vi "Write.vi"(7 "length":u16, 8 "error in (no error)":errorcluster, 9 "Start address":string, 10 "Read Type":variant, 11 "MelsecTCP in":refnum<class "Inovance5UTcp.lvclass">) -> (0 "error out":errorcluster, 3 "MelsecTCP out":refnum<class "Inovance5UTcp.lvclass">)   [LabVIEW 2020, in "HslCommunication.lvlib" / "Inovance5UTcp.lvclass"]
uses:
  Inovance5UTcp.lvclass
  C:/Users/Fred Guo/Desktop/API_Salcomp_CMES/Libraries/HslCommunication/HslCommunication.dll
  HslCommunication.dll
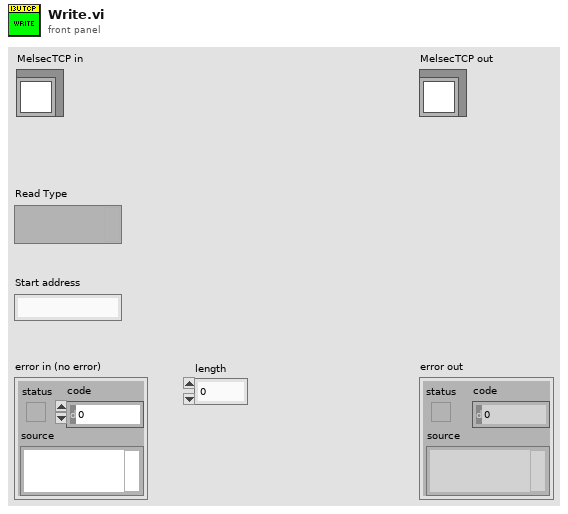
[diagram p1: front panel]
types:
  T1 = typedef "Type Descriptor Enumeration__ogtk.ctl" = enum8{"<Null>", "I8", "I16", "I32", "I64", "U8", "U16", "U32", "U64", "SGL", "DBL", "EXT", "CSG", "CDB", "CXT", "0x0F", "0x10", "0x11", "0x12", "0x13", "0x14", "Enum U8", "Enum U16", "Enum U32", "Enum U64", "SGL PQ", "DBL PQ", "EXT PQ", "CSG PQ", "CDB PQ", "CXT PQ", "0x1F", "0x20", "Boolean", "0x22", "0x23", "0x24", "0x25", "0x26", "0x27", "0x28", "0x29", "0x2A", "0x2B", "0x2C", "0x2D", "0x2E", "0x2F", "String", "0x31", "Path", "Pict", "0x34", "0x35", "0x36", "DAQ", "0x38", "0x39", "0x3A", "0x3B", "0x3C", "0x3D", "0x3E", "0x3F", "Array", "0x41", "0x42", "0x43", "0x44", "0x45", "0x46", "0x47", "0x48", "0x49", "0x4A", "0x4B", "0x4C", "0x4D", "0x4E", "0x4F", "Cluster", "0x51", "0x52", "Variant", "Waveform", "0x55", "0x56", "0x57", "0x58", "0x59", "0x5A", "0x5B", "0x5C", "0x5D", "0x5E", "Fixed Point", "0x60", "0x61", "0x62", "0x63", "0x64", "0x65", "0x66", "0x67", "0x68", "0x69", "0x6A", "0x6B", "0x6C", "0x6D", "0x6E", "0x6F", "Refnum", "0x71", "0x72", "Set Collection", "Map Collection"}
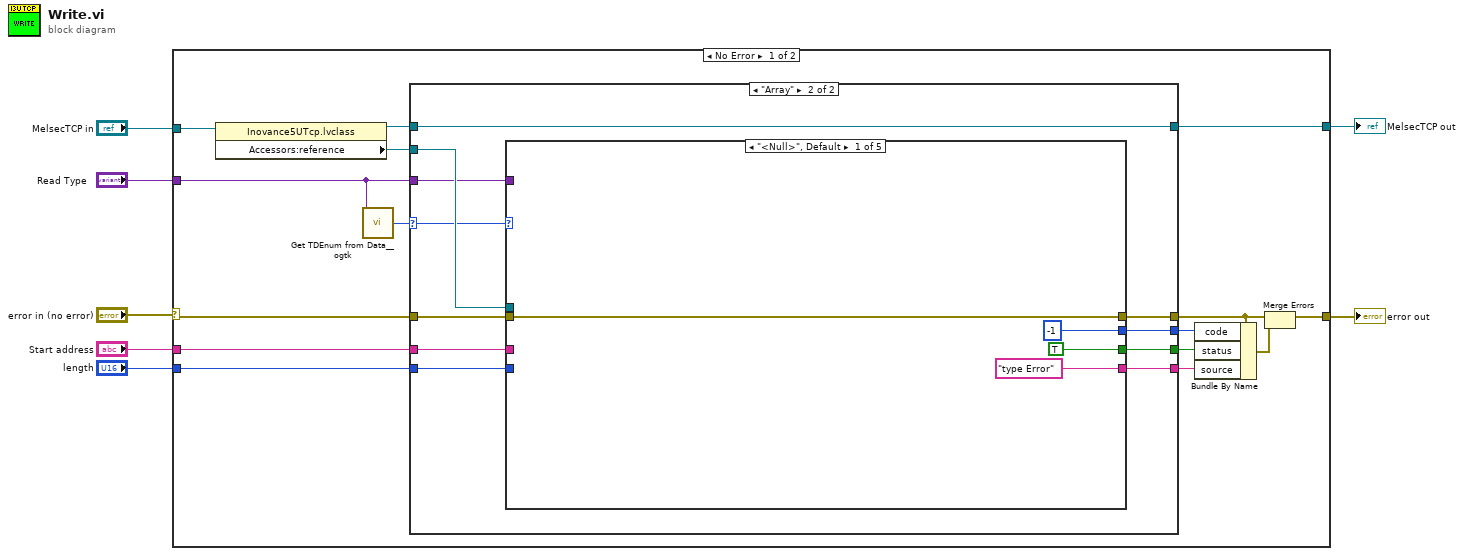
[diagram p0: block diagram]
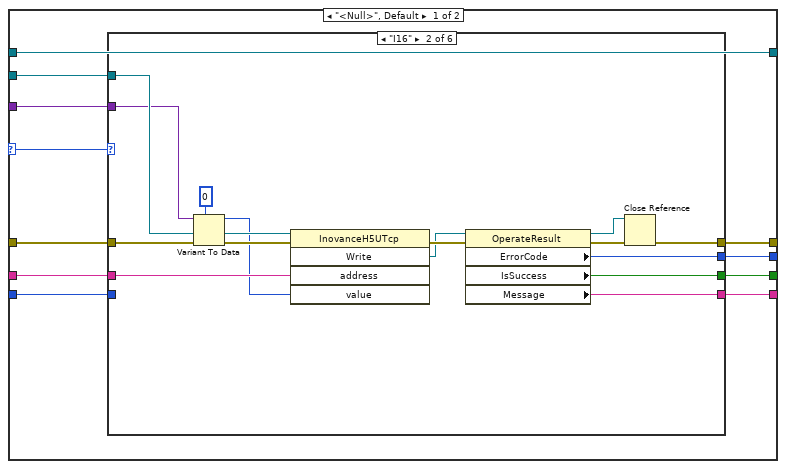
[diagram p2: hidden frame]
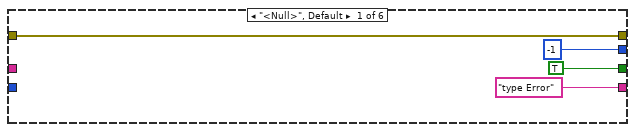
[diagram p3: hidden frame]
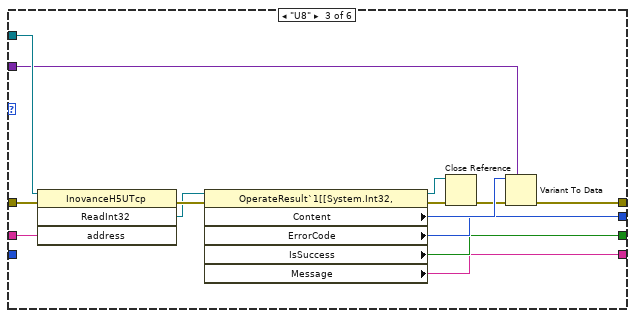
[diagram p4: hidden frame]
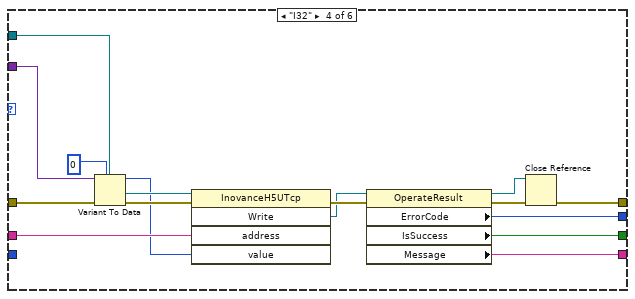
[diagram p5: hidden frame]
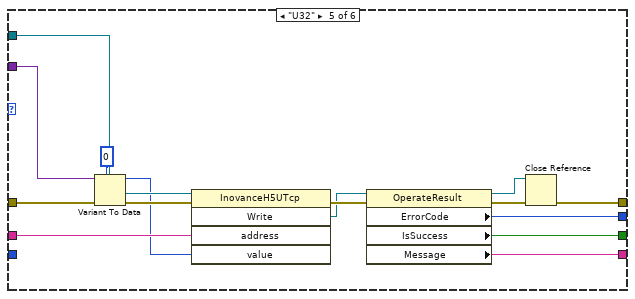
[diagram p6: hidden frame]
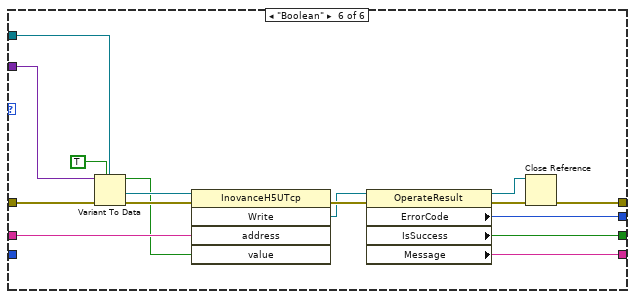
[diagram p7: hidden frame]
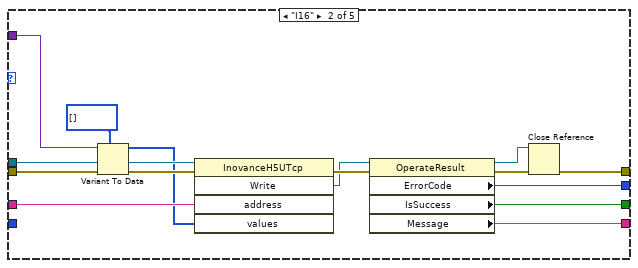
[diagram p8: hidden frame]
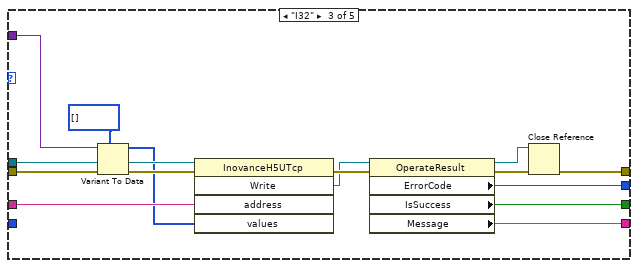
[diagram p9: hidden frame]
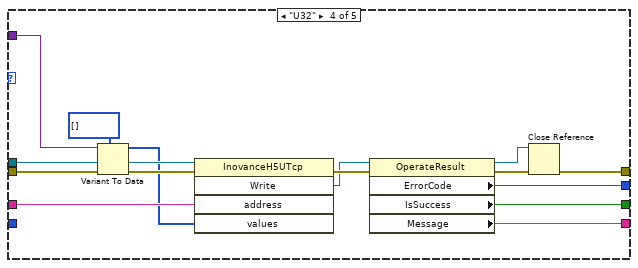
[diagram p10: hidden frame]
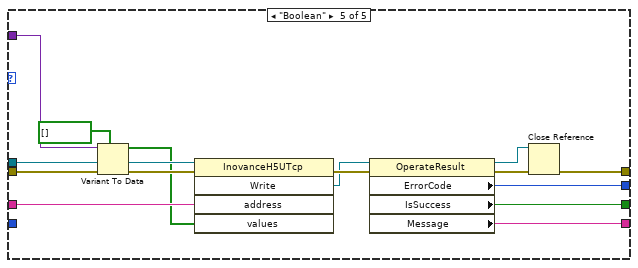
[diagram p11: hidden frame]
diagram:
  n1 = case shown="No Error" "error in (no error)" {
    selector: "error in (no error)" -> [w18 w188]
    tunnel: "MelsecTCP in" -> [w22 w187]
    tunnel: [w8 w187] -> w7
    tunnel: "Start address" -> [w20 _]
    tunnel: [w15 w188] -> w2
    tunnel: "length" -> [w19 _]
    tunnel: "Read Type" -> [w17 _]
    frame No Error {
      n2 = property class="Inovance5UTcp.lvclass"(reference=w22) -> (reference out=w9:refnum<class "Inovance5UTcp.lvclass">, "Accessors:reference"=w21:refnum<k24>)  [unwired: 1 in, 1 out]
      n3 = call <userlib>:"Get TDEnum from Data__ogtk.vi"("Data"=w17) -> ("Type Descriptor Enumeration"=w16:T1)  [unwired: 4 in]
      n4 = case shown="\"Array\"" w16 {
        selector: w16 -> [w27 w116]
        tunnel: w21 -> [w33 w122]
        tunnel: w20 -> [w32 w121]
        tunnel: w19 -> [w31 w120]
        tunnel: w18 -> [w28 w117]
        tunnel: [w30 w119] -> w11
        tunnel: w17 -> [w29 w118]
        tunnel: [w26 w115] -> w14
        tunnel: [w24 w113] -> w12
        tunnel: [w25 w114] -> w13
        tunnel: [w23 w112] -> w8
        tunnel: w9 -> [w23 w112]
        frame "<Null>", Default {
          n5 = case shown="\"I16\"" w27 {
            tunnel: w33 -> [_ w42 w66 w71 w86 w101]
            tunnel: w32 -> [_ w52 w65 w81 w96 w111]
            tunnel: w31 -> [_ _ _ _ _ _]
            tunnel: w28 -> [w37 w51 w64 w80 w95 w110]
            tunnel: [w37 w46 w57 w75 w90 w105] -> w30
            tunnel: [-1 ("ErrorCode") w45 w56 w74 w89 w104] -> w26
            tunnel: [TRUE ("IsSuccess") w44 w55 w73 w88 w103] -> w25
            tunnel: ["type Error" ("Message") w43 w54 w72 w87 w102] -> w24
            tunnel: w29 -> [_ w40 w53 w69 w84 w99]
            frame "<Null>", Default {
            }
            frame "I16" {
              n6 = Variant To Data(error in=w51, type=i16 0, Variant=w40) -> (data=w38:i16, error out=w41:errorcluster)
              n7 = invoke class="InovanceH5UTcp" method="Write"(reference=w42, error in=w41, "address"=w52, "value"=w38) -> (error out=w50:errorcluster, "Write"=w48:refnum<k24>)  [unwired: 1 in, 3 out]
              n8 = property class="OperateResult"(reference=w48, error in=w50) -> (reference out=w47:refnum<k24>, error out=w49:errorcluster, "ErrorCode"=w45:i32, "IsSuccess"=w44:bool, "Message"=w43:string)
              n9 = Close Reference(reference=w47, error in (no error)=w49) -> (error out=w46:errorcluster)
            }
            frame "U8" {
              n10 = invoke class="InovanceH5UTcp" method="ReadInt32"(reference=w66, error in=w64, "address"=w65) -> (error out=w63:errorcluster, "ReadInt32"=w61:refnum<k24>)  [unwired: 1 in, 2 out]
              n11 = property class="OperateResult`1[[System.Int32, "(reference=w61, error in=w63) -> (reference out=w60:refnum<k24>, error out=w62:errorcluster, "Content"=w59:i32, "ErrorCode"=w56:i32, "IsSuccess"=w55:bool, "Message"=w54:string)
              n12 = Close Reference(reference=w60, error in (no error)=w62) -> (error out=w58:errorcluster)
              n13 = Variant To Data(error in=w58, type=w53, Variant=w59) -> (error out=w57:errorcluster)  [unwired: 1 out]
            }
            frame "I32" {
              n14 = Variant To Data(error in=w80, type=0, Variant=w69) -> (data=w67:i32, error out=w70:errorcluster)
              n15 = invoke class="InovanceH5UTcp" method="Write"(reference=w71, error in=w70, "address"=w81, "value"=w67) -> (error out=w79:errorcluster, "Write"=w77:refnum<k24>)  [unwired: 1 in, 3 out]
              n16 = property class="OperateResult"(reference=w77, error in=w79) -> (reference out=w76:refnum<k24>, error out=w78:errorcluster, "ErrorCode"=w74:i32, "IsSuccess"=w73:bool, "Message"=w72:string)
              n17 = Close Reference(reference=w76, error in (no error)=w78) -> (error out=w75:errorcluster)
            }
            frame "U32" {
              n18 = Variant To Data(error in=w95, type=u32 0, Variant=w84) -> (data=w82:u32, error out=w85:errorcluster)
              n19 = invoke class="InovanceH5UTcp" method="Write"(reference=w86, error in=w85, "address"=w96, "value"=w82) -> (error out=w94:errorcluster, "Write"=w92:refnum<k24>)  [unwired: 1 in, 3 out]
              n20 = property class="OperateResult"(reference=w92, error in=w94) -> (reference out=w91:refnum<k24>, error out=w93:errorcluster, "ErrorCode"=w89:i32, "IsSuccess"=w88:bool, "Message"=w87:string)
              n21 = Close Reference(reference=w91, error in (no error)=w93) -> (error out=w90:errorcluster)
            }
            frame "Boolean" {
              n22 = Variant To Data(error in=w110, type=TRUE, Variant=w99) -> (data=w97:bool, error out=w100:errorcluster)
              n23 = invoke class="InovanceH5UTcp" method="Write"(reference=w101, error in=w100, "address"=w111, "value"=w97) -> (error out=w109:errorcluster, "Write"=w107:refnum<k24>)  [unwired: 1 in, 3 out]
              n24 = property class="OperateResult"(reference=w107, error in=w109) -> (reference out=w106:refnum<k24>, error out=w108:errorcluster, "ErrorCode"=w104:i32, "IsSuccess"=w103:bool, "Message"=w102:string)
              n25 = Close Reference(reference=w106, error in (no error)=w108) -> (error out=w105:errorcluster)
            }
          }
        }
        frame "Array" {
          n26 = case shown="\"<Null>\", Default" w116 {
            tunnel: w122 -> [_ w131 w146 w161 w176]
            tunnel: w121 -> [_ w141 w156 w171 w186]
            tunnel: w120 -> [_ _ _ _ _]
            tunnel: w117 -> [w126 w140 w155 w170 w185]
            tunnel: [w126 w135 w150 w165 w180] -> w119
            tunnel: [-1 ("ErrorCode") w134 w149 w164 w179] -> w115
            tunnel: [TRUE ("IsSuccess") w133 w148 w163 w178] -> w114
            tunnel: ["type Error" ("Message") w132 w147 w162 w177] -> w113
            tunnel: w118 -> [_ w129 w144 w159 w174]
            frame "<Null>", Default {
            }
            frame "I16" {
              n27 = Variant To Data(error in=w140, type=i16[] [], Variant=w129) -> (data=w127:i16[], error out=w130:errorcluster)
              n28 = invoke class="InovanceH5UTcp" method="Write"(reference=w131, error in=w130, "address"=w141, "values"=w127) -> (error out=w139:errorcluster, "Write"=w137:refnum<k24>)  [unwired: 1 in, 3 out]
              n29 = property class="OperateResult"(reference=w137, error in=w139) -> (reference out=w136:refnum<k24>, error out=w138:errorcluster, "ErrorCode"=w134:i32, "IsSuccess"=w133:bool, "Message"=w132:string)
              n30 = Close Reference(reference=w136, error in (no error)=w138) -> (error out=w135:errorcluster)
            }
            frame "I32" {
              n31 = Variant To Data(error in=w155, type=i32[] [], Variant=w144) -> (data=w142:i32[], error out=w145:errorcluster)
              n32 = invoke class="InovanceH5UTcp" method="Write"(reference=w146, error in=w145, "address"=w156, "values"=w142) -> (error out=w154:errorcluster, "Write"=w152:refnum<k24>)  [unwired: 1 in, 3 out]
              n33 = property class="OperateResult"(reference=w152, error in=w154) -> (reference out=w151:refnum<k24>, error out=w153:errorcluster, "ErrorCode"=w149:i32, "IsSuccess"=w148:bool, "Message"=w147:string)
              n34 = Close Reference(reference=w151, error in (no error)=w153) -> (error out=w150:errorcluster)
            }
            frame "U32" {
              n35 = Variant To Data(error in=w170, type=u32[] [], Variant=w159) -> (data=w157:u32[], error out=w160:errorcluster)
              n36 = invoke class="InovanceH5UTcp" method="Write"(reference=w161, error in=w160, "address"=w171, "values"=w157) -> (error out=w169:errorcluster, "Write"=w167:refnum<k24>)  [unwired: 1 in, 3 out]
              n37 = property class="OperateResult"(reference=w167, error in=w169) -> (reference out=w166:refnum<k24>, error out=w168:errorcluster, "ErrorCode"=w164:i32, "IsSuccess"=w163:bool, "Message"=w162:string)
              n38 = Close Reference(reference=w166, error in (no error)=w168) -> (error out=w165:errorcluster)
            }
            frame "Boolean" {
              n39 = Variant To Data(error in=w185, type=bool[] [], Variant=w174) -> (data=w172:bool[], error out=w175:errorcluster)
              n40 = invoke class="InovanceH5UTcp" method="Write"(reference=w176, error in=w175, "address"=w186, "values"=w172) -> (error out=w184:errorcluster, "Write"=w182:refnum<k24>)  [unwired: 1 in, 3 out]
              n41 = property class="OperateResult"(reference=w182, error in=w184) -> (reference out=w181:refnum<k24>, error out=w183:errorcluster, "ErrorCode"=w179:i32, "IsSuccess"=w178:bool, "Message"=w177:string)
              n42 = Close Reference(reference=w181, error in (no error)=w183) -> (error out=w180:errorcluster)
            }
          }
        }
      }
      n43 = Bundle By Name(cluster=w11, "code"=w14, "status"=w13, "source"=w12) -> (w10:errorcluster)
      n44 = Merge Errors(w11, w10) -> (w15:errorcluster)
    }
    frame Error {
    }
  }
  "error out" <- w2
  "MelsecTCP out" <- w7
